vi "Position.vi"(5 "Username":string, 6 "Password":string, 7 "Address":string, 8 "Error In":errorcluster) -> (0 "Error Out":errorcluster)   [LabVIEW 2018, in "Tests.lvlib" / "SFTP File.lvlib"]
uses:
  SFTP File.lvlib
  src/Toolkit/API/SFTP File/API/Typedefs/Flags.ctl
  src/Toolkit/API/SFTP File/SFTP File.lvclass/SFTP File.ctl
  src/Toolkit/API/SFTP/SFTP.lvclass/SFTP.ctl
  src/Toolkit/API/SFTP/Utility/Read Shared Library.vi
  src/Toolkit/API/Session/Utility/Read Shared Library.vi
  src/Toolkit/Support/Check Status.vi
  <vilib>/addons/_JKI Toolkits/Caraya/classes/Test/Test.lvclass
  <vilib>/addons/_JKI Toolkits/Caraya/classes/Assert/Assert.lvclass
  src/Toolkit/API/SFTP File/SFTP File.lvclass
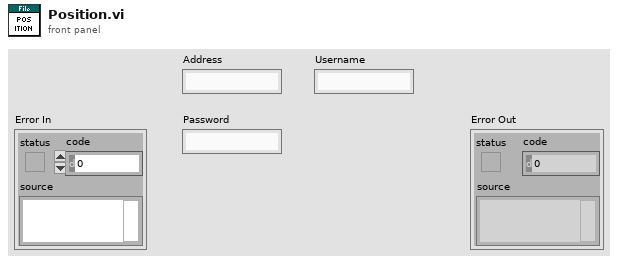
[diagram p1: front panel]
types:
  T1 = typedef "Toolkit.lvlib/SFTP File.lvclass/Flags.ctl" = cluster{"Read":bool, "Write":bool, "Append":bool, "Create":bool, "Truncate":bool, "Exclude":bool}
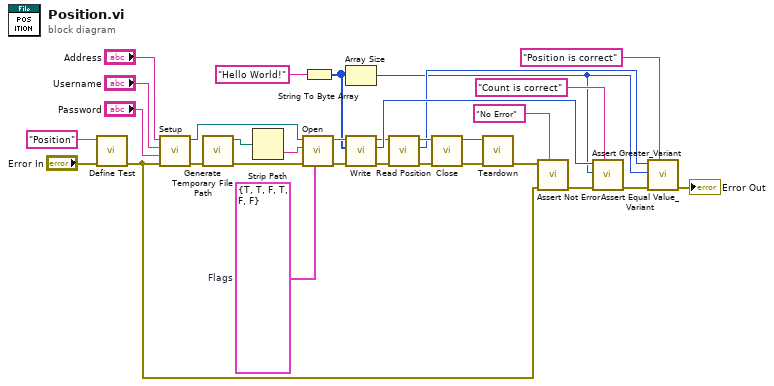
[diagram p0: block diagram]
diagram:
  w9 = T1 {"Read"=TRUE, "Write"=TRUE, "Append"=FALSE, "Create"=TRUE, "Truncate"=FALSE, "Exclude"=FALSE}  # Flags
  n1 = call <vilib>:"Define Test.vi"("error in (no error)"="Error In", "Label (VI Title)"="Position") -> ("error out"=w23:errorcluster)  [unwired: 9 in]
  n2 = call "Setup.vi"("Error In"=w23, "Password"="Password", "Username"="Username", "Address"="Address") -> ("Error Out"=w18:errorcluster, "SFTP"=w20:refnum<class "SFTP.lvclass">)  [unwired: 6 in]
  n3 = call <vilib>:"Generate Temporary File Path.vi"("error in (no error)"=w18) -> ("error out"=w17:errorcluster, "Unique Temporary File Path"=w16:path)  [unwired: 9 in]
  n4 = Strip Path(path=w16) -> (name=w15:string)  [unwired: 1 out]
  n5 = call "Open.vi"("Flags"=w9, "Error In"=w17, "Remote Path"=w15, "SFTP"=w20) -> ("Error Out"=w12:errorcluster, "SFTP File"=w14:refnum<class "SFTP File.lvclass">)  [unwired: 6 in]
  n6 = String To Byte Array(string="Hello World!") -> (unsigned byte array=w10:u8[])
  n7 = Array Size(array=w10) -> (size(s)=w2:i32)
  n8 = call "Write.vi"("Error In"=w12, "Data"=w10, "SFTP File In"=w14) -> ("Error Out"=w5:errorcluster, "Count"=w13:i64, "SFTP File Out"=w8:refnum<class "SFTP File.lvclass">)  [unwired: 6 in]
  n9 = call "Read Position.vi"("Error In"=w5, "SFTP File In"=w8) -> ("Error Out"=w6:errorcluster, "Position"=w3:u64, "SFTP File Out"=w7:refnum<class "SFTP File.lvclass">)  [unwired: 7 in]
  n10 = call "Close.vi"("Error In"=w6, "SFTP File"=w7) -> ("Error Out"=w22:errorcluster, "SFTP"=w19:refnum<class "SFTP.lvclass">)  [unwired: 8 in]
  n11 = call "Teardown.vi"("Error In"=w22, "SFTP"=w19) -> ("Error Out"=w21:errorcluster)  [unwired: 9 in]
  n12 = call <vilib>:"Assert Not Error.vi"("Label"="No Error", "error in (no error)"=w23, "Not Error?"=w21) -> ("error out"=w29:errorcluster)  [unwired: 8 in]
  n13 = call <vilib>:"Assert Greater_Variant.vi"("Label"="Count is correct", "error in (no error)"=w29, "Y"=w2, "X"=w13) -> ("error out"=w28:errorcluster)  [unwired: 7 in]
  n14 = call <vilib>:"Assert Equal Value_Variant.vi"("Label"="Position is correct", "error in (no error)"=w28, "Y"=w2, "X"=w3) -> ("error out"=→"Error Out":errorcluster)  [unwired: 7 in]
